vi "svfa_Check Multi Tone Detection Iteration Condition.vi"(2 "precision":dbl format="%.2e", 3 "peaks before":T1(array[cluster]) {"phase [degree]" format="%.2f"; "amplitude" format="%.2f"; "frequency [Hz]" format="%.2f"}, 4 "peaks after":T1(array[cluster]) {"phase [degree]" format="%.2f"; "amplitude" format="%.2f"; "frequency [Hz]" format="%.2f"}) -> (0 "stable?":bool[](array[boolean]), 1 "all stable?":bool)   [LabVIEW 2017]
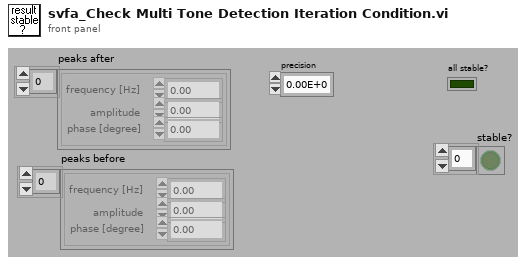
[diagram p1: front panel]
types:
  T1 = cluster{"frequency [Hz]":dbl, "amplitude":dbl, "phase [degree]":dbl}[]
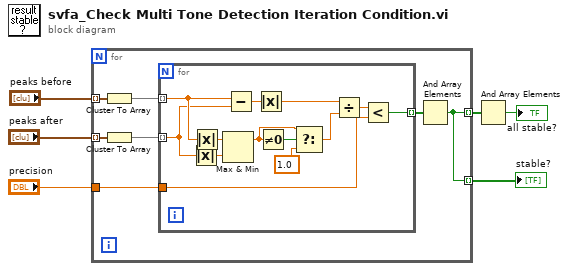
[diagram p0: block diagram]
diagram:
  n1 = for {
    tunnel: "peaks before" -> [w13] mode=indexing
    tunnel: "peaks after" -> [w12] mode=indexing
    tunnel: [w8] -> w4 mode=indexing
    tunnel: [w8] -> w2 mode=indexing
    tunnel: "precision" -> [w7]
    n2 = Cluster To Array(cluster=w13) -> (array=w11:dbl[])
    n3 = Cluster To Array(cluster=w12) -> (array=w10:dbl[])
    n4 = for {
      tunnel: w11 -> [w21] mode=indexing
      tunnel: w10 -> [w20] mode=indexing
      tunnel: [w15] -> w9 mode=indexing
      tunnel: w7 -> [w14]
      n5 = Absolute Value(x=w20) -> (abs(x)=w25:dbl)
      n6 = Absolute Value(x=w21) -> (abs(x)=w26:dbl)
      n7 = Max & Min(x=w26, y=w25) -> (max(x,y)=w23:dbl)  [unwired: 1 out]
      n8 = Subtract(x=w21, y=w20) -> (x-y=w19:dbl)
      n9 = Absolute Value(x=w19) -> (abs(x)=w18:dbl)
      n10 = Not Equal To 0?(x=w23) -> (x != 0?=w24:bool)
      n11 = Select(t=w23, s=w24, f=1.0) -> (s? t:f=w17:dbl)
      n12 = Divide(x=w18, y=w17) -> (x/y=w16:dbl)
      n13 = Less?(x=w16, y=w14) -> (x < y?=w15:bool)
    }
    n14 = And Array Elements(Boolean array=w9) -> (logical AND=w8:bool)
  }
  "stable?" <- w2
  n15 = And Array Elements(Boolean array=w4) -> (logical AND=→"all stable?":bool)
